vi "Set-Get Histogram Min & Max Cursor Locations.vi"(4 "Upper Percentile [0-100], Default: 95":dbl=95.0 min=0.0 max=100.0, 6 "Lower Percentile [0-100], Default: 5":dbl=5.0 min=0.0 max=100.0, 8 "error in (no error)":errorcluster, 9 "Set/Get (F) Contrast":bool, 10 "XYGraph in":refnum<vi>, 11 "Histogram":cluster{"Axis":dbl[], "Histogram":dbl[]}) -> (0 "error out":errorcluster, 1 "Min Location":dbl, 2 "Max Location":dbl)   [LabVIEW 2021, in "Histograms.lvlib"]
uses:
  Histograms.lvlib
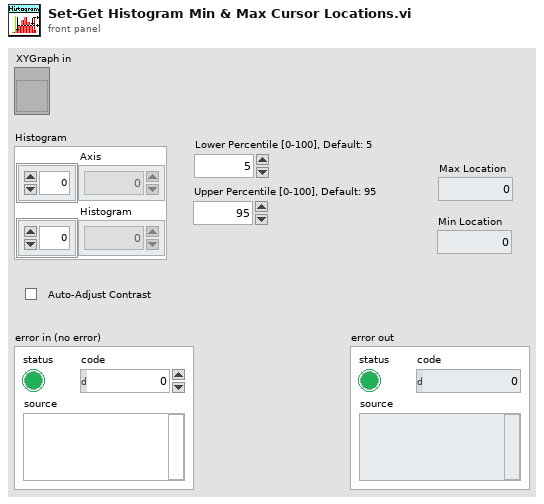
[diagram p1: front panel]
types:
  T1 = typedef "LVCursorListTypeDef.ctl" = cluster{"Name":string, "Color":u32, "Style":u8, "Point Style":u8, "Name Visible":bool, "Allow Drag":bool, "Cursor Mode":u32, "Plot":i32, "Index":i32, "Position":cluster{"X":dbl, "Y":dbl}, "X Scale":u32, "Y Scale":u32, "Watch Plots":i32[], "Watch All Plots":bool, "Plot Area":i32, "Label Offset":cluster{"X":dbl, "Y":dbl}}[]
  T2 = cluster{"Name":string, "Color":u32, "Style":u8, "Point Style":u8, "Name Visible":bool, "Allow Drag":bool, "Cursor Mode":u32, "Plot":i32, "Index":i32, "Position":cluster{"X":dbl, "Y":dbl}, "X Scale":u32, "Y Scale":u32, "Watch Plots":i32[], "Watch All Plots":bool, "Plot Area":i32, "Label Offset":cluster{"X":dbl, "Y":dbl}}
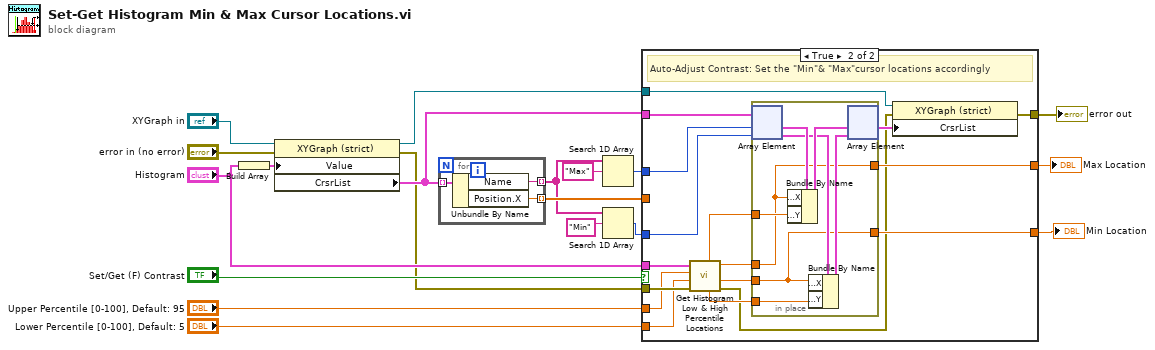
[diagram p0: block diagram]
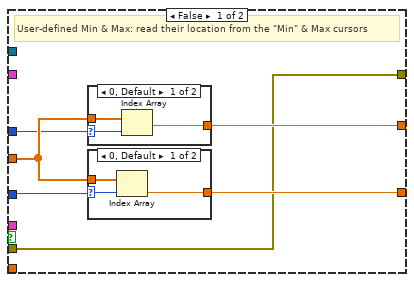
[diagram p2: hidden frame]
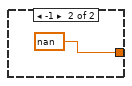
[diagram p3: hidden frame]
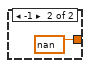
[diagram p4: hidden frame]
diagram:
  n1 = Build Array("Histogram") -> (w10:cluster{"Axis":dbl[], "Histogram":dbl[]}[])
  n2 = property class="XYGraph (strict)"(reference="XYGraph in", error in="error in (no error)", "Value"=w10) -> (reference out=w5:refnum<vi>, error out=w4:errorcluster, "CrsrList"=w6:T1)
  n3 = for {
    tunnel: w6 -> [w22] mode=indexing
    tunnel: [w21] -> w12 mode=indexing
    tunnel: [w20] -> w16 mode=indexing
    n4 = Unbundle By Name(w22) -> ("Name"=w21:string, "Position.X"=w20:dbl)
  }
  n5 = Search 1D Array(1D array=w12, element="Max") -> (index of element=w14:i32)  [unwired: 1 in]
  n6 = Search 1D Array(1D array=w12, element="Min") -> (index of element=w15:i32)  [unwired: 1 in]
  n7 = case shown="True" "Set/Get (F) Contrast" {
    tunnel: [w28 w49] -> w18
    tunnel: [w27 w48] -> w17
    tunnel: w16 -> [w26 _]
    tunnel: w15 -> [w25 w51]
    tunnel: w14 -> [w24 w52]
    tunnel: "Histogram" -> [_ w53]
    tunnel: w6 -> [_ w37]
    tunnel: w5 -> [_ w46]
    tunnel: w4 -> [w23 w41]
    tunnel: [w23 w47] -> w3
    tunnel: "Upper Percentile [0-100], Default: 95" -> [_ w40]
    tunnel: "Lower Percentile [0-100], Default: 5" -> [_ w39]
    frame False {
      # "User-defined Min & Max: read their location from the \"Min\" & Max cursors"
      n8 = case shown="0, Default" w24 {
        selector: w24 -> [w34 _]
        tunnel: w26 -> [w35 _]
        tunnel: [w33 nan ("X")] -> w28
        frame 0, Default {
          n9 = Index Array(array=w35, index=w34) -> (element=w33:dbl)
        }
        frame -1 {
        }
      }
      n10 = case shown="0, Default" w25 {
        selector: w25 -> [w30 _]
        tunnel: w26 -> [w31 _]
        tunnel: [w29 nan ("X")] -> w27
        frame 0, Default {
          n11 = Index Array(array=w31, index=w30) -> (element=w29:dbl)
        }
        frame -1 {
        }
      }
    }
    frame True {
      # "Auto-Adjust Contrast: Set the \"Min\"& \"Max\"cursor locations accordingly"
      n12 = call "Get Histogram Low & High Percentile Locations.vi"("Error In"=w41, "Lower Percentile [0-100], Default: 5"=w39, "Upper Percentile [0-100], Default: 95"=w40, "Histogram"=w53) -> ("Error Out"=w38:errorcluster, "Lower Percentile Location"=w43:dbl, "Upper Percentile Location"=w45:dbl, "Lower Percentile Bin"=w42:dbl, "Upper Percentile Bin"=w44:dbl)  [unwired: 3 in]
      n13 = in-place {
        in-place-border: w45 -> [w55]
        in-place-border: w44 -> [w59]
        in-place-border: w42 -> [w58]
        in-place-border: w43 -> [w54]
        in-place-border: [w55] -> w49
        in-place-border: [w54] -> w48
        n14 = in-place-array #1(w37, w52, w51) -> (w61:T2, w57:T2)
        n15 = Bundle By Name(cluster=w61, "Position.X"=w55, "Position.Y"=w59) -> (w60:T2)
        n16 = Bundle By Name(cluster=w57, "Position.X"=w54, "Position.Y"=w58) -> (w56:T2)
        n17 = in-place-array #1(w60, w56) -> (w50:T1)  [unwired: 2 out]
      }
      n18 = property class="XYGraph (strict)"(reference=w46, error in=w38, "CrsrList"=w50) -> (error out=w47:errorcluster)  [unwired: 1 out]
    }
  }
  "error out" <- w3
  "Max Location" <- w18
  "Min Location" <- w17
